vi "Find Enemies.vi"(11 "Square":refnum<class "Square.lvclass">) -> (1 "Any Enemies?":bool, 2 "Enemy Directions":T1[](array[typedef]))   [LabVIEW 2020, in "SquareBattle.lvlib" / "Square.lvclass"]
uses:
  Square.lvclass
  Direction.ctl
  Square.lvclass/Square.ctl
  SquareBattle.lvlib
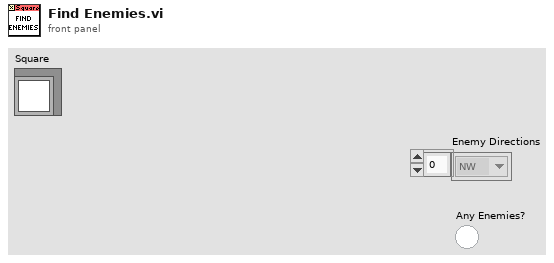
[diagram p1: front panel]
types:
  T1 = typedef "SquareBattle.lvlib/Direction.ctl" = enum16{"NW", "N", "NE", "E", "SE", "S", "SW", "W"}
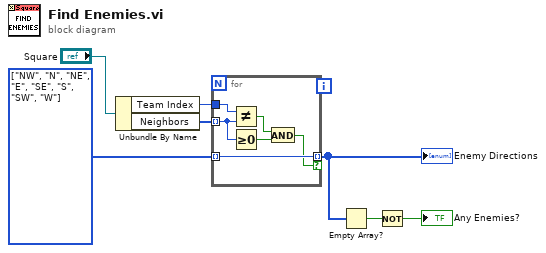
[diagram p0: block diagram]
diagram:
  w4 = T1[] [enum."NW", enum."N", enum."NE", enum."E", enum."SE", enum."S", enum."SW", enum."W"] items=["NW", "N", "NE", "E", "SE", "S", "SW", "W"] ("Enemy Directions")
  n1 = Unbundle By Name("Square") -> ("Team Index"=w6:i32, "Neighbors"=w5:i32[])
  n2 = for {
    tunnel: w6 -> [w12]
    tunnel: w5 -> [w11] mode=indexing
    tunnel: w4 -> [w13] mode=indexing
    tunnel: [w13] -> w3 mode=indexing if=w8
    n3 = Not Equal?(x=w12, y=w11) -> (x != y?=w9:bool)
    n4 = Greater Or Equal To 0?(x=w11) -> (x >= 0?=w10:bool)
    n5 = And(x=w9, y=w10) -> (x .and. y?=w8:bool)
  }
  "Enemy Directions" <- w3
  n6 = Empty Array?(array=w3) -> (empty?=w2:bool)
  n7 = Not(x=w2) -> (.not. x?=→"Any Enemies?":bool)
